vi "String Paths - Common Base Folder.vi"(5 "error IN":errorcluster, 7 "Data File FULL Paths":string[](array[string])) -> (11 "Common Base path depth":i32, 13 "Commom base Path":path, 19 "error OUT":errorcluster)   [LabVIEW 2020, in "Generic Utilities.lvclass"]
uses:
  Generic Utilities.lvclass
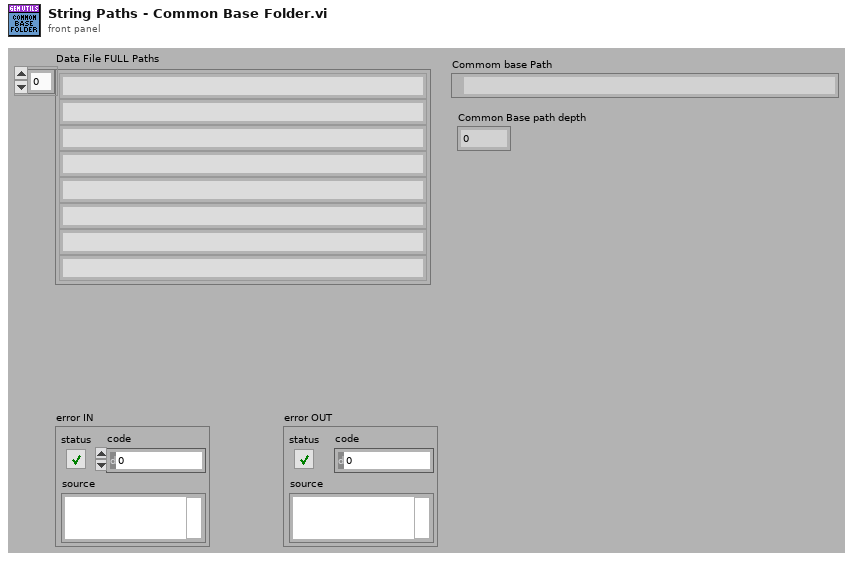
[diagram p1: front panel]
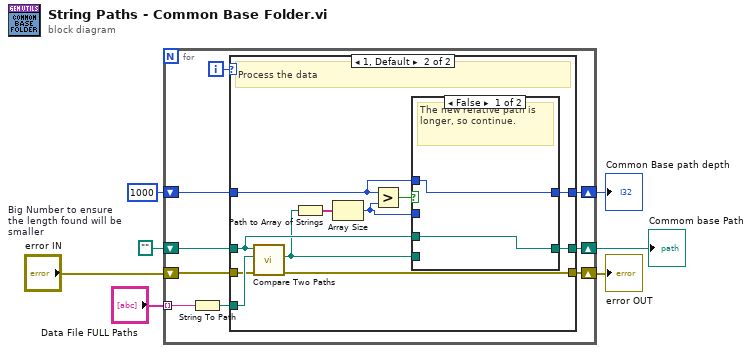
[diagram p0: block diagram]
diagram:
  w5 = 1000  # Big Number to ensure the length found will be smaller
  n1 = for {
    tunnel: "Data File FULL Paths" -> [w16] mode=indexing
    shift-right: [w14] -> w7
    shift-left: path "" -> [w12]
    shift-right: [w11] -> w4
    shift-left: "error IN" -> [w10]
    shift-right: [w9] -> w6
    shift-left: w5 -> [w8]
    i -> [w15]
    n2 = String To Path(string=w16) -> (path=w13:path)
    n3 = case shown="1, Default" w15 {
      tunnel: [w19 w23] -> w14
      tunnel: w13 -> [w19 w30]
      tunnel: w12 -> [_ w22]
      tunnel: [w18 w29] -> w11
      tunnel: w10 -> [w18 w28]
      tunnel: [w17 w25] -> w9
      tunnel: w8 -> [w17 w24]
      frame 0 {
        # "Initilize the shift register with the first valid values."
      }
      frame 1, Default {
        # "Process the data"
        n4 = call <vilib>:"Compare Two Paths.vi"("error in (no error)"=w28, "Path 2"=w30, "Path 1"=w22) -> ("error out"=w29:errorcluster, "Common Path"=w20:path)  [unwired: 5 in, 2 out]
        n5 = Path to Array of Strings(0:w20) -> (2:w27:string[])  [unwired: 1 out]
        n6 = Array Size(array=w27) -> (size(s)=w21:i32)
        n7 = Greater?(x=w24, y=w21) -> (0:w26:bool)
        n8 = case shown="False" w26 {
          tunnel: [w32 w34] -> w25
          tunnel: w24 -> [w32 _]
          tunnel: [w31 w33] -> w23
          tunnel: w22 -> [w31 _]
          tunnel: w21 -> [_ w34]
          tunnel: w20 -> [_ w33]
          frame False {
            # "The new relative path is longer, so continue."
          }
          frame True {
            # "The new relative path is shorter, so keep it"
          }
        }
      }
    }
  }
  "error OUT" <- w4
  "Common Base path depth" <- w6
  "Commom base Path" <- w7
